vi "ProcessState-Running.vi"(3 "ProcessStateNotifier in":refnum<notifier>, 9 "error in (no error)":errorcluster) -> (0 "ProcessStateNotifier out":refnum<notifier>, 6 "error out":errorcluster)   [LabVIEW 2009]
uses:
  ProcessState.ctl
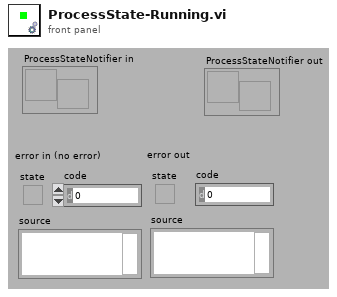
[diagram p1: front panel]
types:
  T1 = typedef "ProcessState.ctl" = enum16{"STARTING", "RUNNING", "STOPPING", "STOPPPED"}
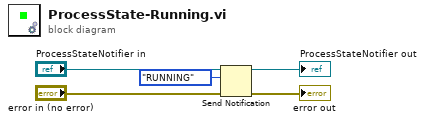
[diagram p0: block diagram]
diagram:
  n1 = Send Notification(notification=ProcessState."RUNNING", notifier="ProcessStateNotifier in", error in (no error)="error in (no error)") -> (notifier out=→"ProcessStateNotifier out":refnum<notifier>, error out=→"error out":errorcluster)
